vi "수신vi.vi"() -> ()   [LabVIEW 2014]
uses:
  <vilib>/Utility/tcp.llb/UDP Multicast Read-Only Open.vi
panel:
  out "웨이브폼 그래프":dbl[](graph)
  in  "정지":bool
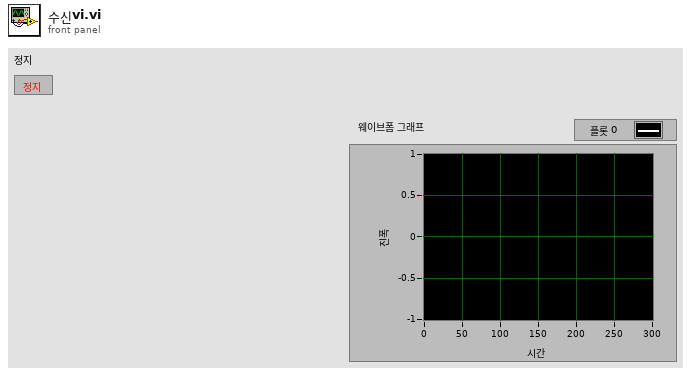
[diagram p1: front panel]
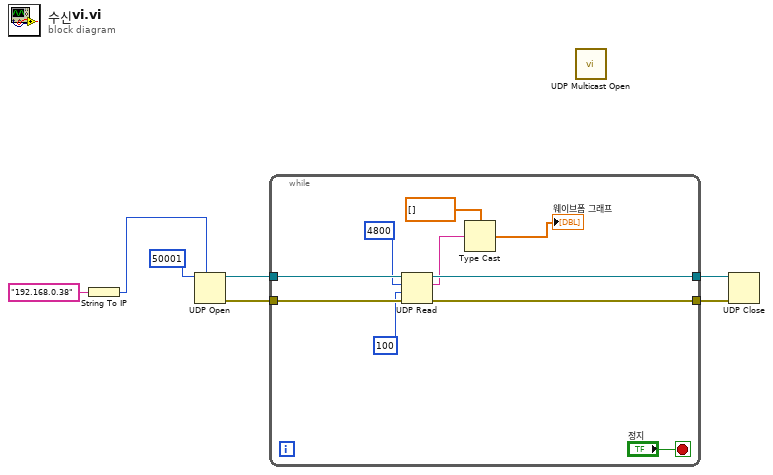
[diagram p0: block diagram]
diagram:
  n1 = String To IP(1:"192.168.0.38" ("이름")) -> (0:w1:u32)
  n2 = UDP Open(7:w1, 11:u16 50001 ("포트")) -> (port=w6:refnum<k16>, 0:w5:errorcluster)  [unwired: 3 in, 1 out]
  n3 = while {
    tunnel: w6 -> [w16]
    tunnel: w5 -> [w15]
    tunnel: [w14] -> w4
    tunnel: [w13] -> w3
    stop <- "정지" stop-if-true
    n4 = UDP Read(connection ID=w16, max size (548)=4800 ("최대 크기(548)"), timeout ms (25000)=100 ("타임아웃 ms (25000)"), 8:w15) -> (data out=w10:string, error out=w13:errorcluster, 3:w14:refnum<k16>)  [unwired: 2 out]
    n5 = Type Cast(type=dbl[] [] ("웨이브폼 그래프 2"), x=w10) -> (*(type *) &x=→"웨이브폼 그래프":dbl[])
  }
  n6 = call-poly <vilib>:"UDP Multicast Open.vi"() -> ()  [unwired: 9 in, 3 out]
  n7 = UDP Close(connection ID=w4, 8:w3) -> ()  [unwired: 2 out]
